vi "Compression.vi"(5 "measure call context in":refnum<class "Measure Call Context.lvclass">, 7 "SMU Settings":T2={"SMU Name"="PXI1Slot15", "SMU Channel"="2", "IDD Current Limit (A)"=0.0}, 8 "error in":errorcluster, 9 "RFmx Settings":T3={"RFmx Name"="5842_0", "RFmx Port"="", "Attenuation"={"Mode"=enum."Constant Attenuation", "Constant Attenuation"={"RFmx External Attenuation (dB)"=1.2}, "s2p File"={"RFmx S-Parameters Orientation"=24000, "RFmx Attenuation s2p File"=path ""}}} {"Attenuation"."s2p File"."RFmx S-Parameters Orientation" items=["Port1 Towards DUT"=24000, "Port2 Towards DUT"=24001]; "Attenuation"."Constant Attenuation"."RFmx External Attenuation (dB)" format="%.2f"}, 10 "RFSG Settings":T4={"RFSG Name"="5842_0", "RFSG Port"="", "Attenuation"={"Mode"=enum."Constant Attenuation", "Contant Attenuation"={"RFSG External Attenuation (dB)"=2.0}, "s2p File"={"RFSG S-parameters Orientation"=24000, "RFSG s2p File Path"=path ""}}} {"Attenuation"."s2p File"."RFSG S-parameters Orientation" items=["Port1 Towards DUT"=24000, "Port2 Towards DUT"=24001]; "Attenuation"."Contant Attenuation"."RFSG External Attenuation (dB)" format="%.2f"}, 11 "Test Configuration":T5={"Expected DUT Gain (dB)"=17.5, "Max Linear Range (dBm)"=-10.0, "Compression Point (dB)"=1.0, "Pout at Pin (dBm)"=1.0, "RFSG Frequency Start (Hz)"=6000000000.0, "RFSG Frequency Stop (Hz)"=18000000000.0, "RFSG Number of Frequency Step"=10, "Power Start (dBm)"=-20.0, "Power Stop(dBm)"=1.0, "Power Step Size (dB)"=4.0, "RBW (Hz)"=5000000.0, "Modes"={"RF Measurement Interval (s)"=0.001, "DC Measurement Interval (s)"=0.0, "Power Stimulus Mode"=enum."Constant Power and RF", "CP_CW_DC Source Delay (s)"=0.0002, "CP_PRF_RF Pulse Width (s)"=0.0009, "CP_PRF_PRI (s)"=0.015, "CP_PRF_DC Source Delay (s)"=0.0, "CP_PRF_RFmx Trigger Delay (s)"=0.2, "PP_PRF_RF Pulse Width (s)"=0.0, "PP_PRF_PRI (s)"=0.0, "PP_PRF_DC Pulse Width (s)"=0.0008, "PP_PRF_Bias Voltage Level (V)"=0.0, "PP_PRF_Bias Current Limit (A)"=0.2, "PP_PRF_DC Source Delay (s)"=0.0, "PP_PRF_RFmx Trigger Delay (s)"=0.0}} {"Pout at Pin (dBm)" format="%#pdBm"; "Modes"."PP_PRF_RFmx Trigger Delay (s)" format="%#ps"; "Modes"."PP_PRF_DC Source Delay (s)" format="%#ps"; "Modes"."PP_PRF_Bias Current Limit (A)" format="%#pA"; "Modes"."PP_PRF_Bias Voltage Level (V)" format="%#pV"; "Modes"."PP_PRF_DC Pulse Width (s)" format="%#ps"; "Modes"."PP_PRF_PRI (s)" format="%#ps"; "Modes"."PP_PRF_RF Pulse Width (s)" format="%#ps"; "Modes"."CP_PRF_RFmx Trigger Delay (s)" format="%#ps"; "Modes"."CP_PRF_DC Source Delay (s)" format="%#ps"; "Modes"."CP_PRF_PRI (s)" format="%#ps"; "Modes"."CP_PRF_RF Pulse Width (s)" format="%#ps"; "Modes"."CP_CW_DC Source Delay (s)" format="%#ps"; "Modes"."DC Measurement Interval (s)" format="%#_6p"; "RFSG Frequency Stop (Hz)" format="%#_6p"; "Power Start (dBm)" format="%#_6p"; "Power Stop(dBm)" format="%#_6p"; "RFSG Frequency Start (Hz)" format="%#_6p"; "Expected DUT Gain (dB)" step=1.0 format="%#_6p"}) -> (0 "error out":errorcluster, 3 "Data":T1)   [LabVIEW 2023]
doc: "This example demonstrates how to use MMICsc API for performing PAE measurements and calibration"
uses:
  Controls/Test Config - Compression.ctl
  Controls/RFSG Config - Compression.ctl
  Controls/RFmx Config - Compression.ctl
  <vilib>/Plug-In SDKs/Measurements/Measure Call Context/Measure Call Context.lvclass
  Controls/SMU Config - Compression.ctl
  Controls/Results - Compression.ctl
  <vilib>/niPAEML/Commit Measurement.vi
  <vilib>/niPAEML/Commit NIDCPower.vi
  <vilib>/niPAEML/PAE Measurement.lvlib
panel:
  out "voltage measurements":dbl[](array[numeric])
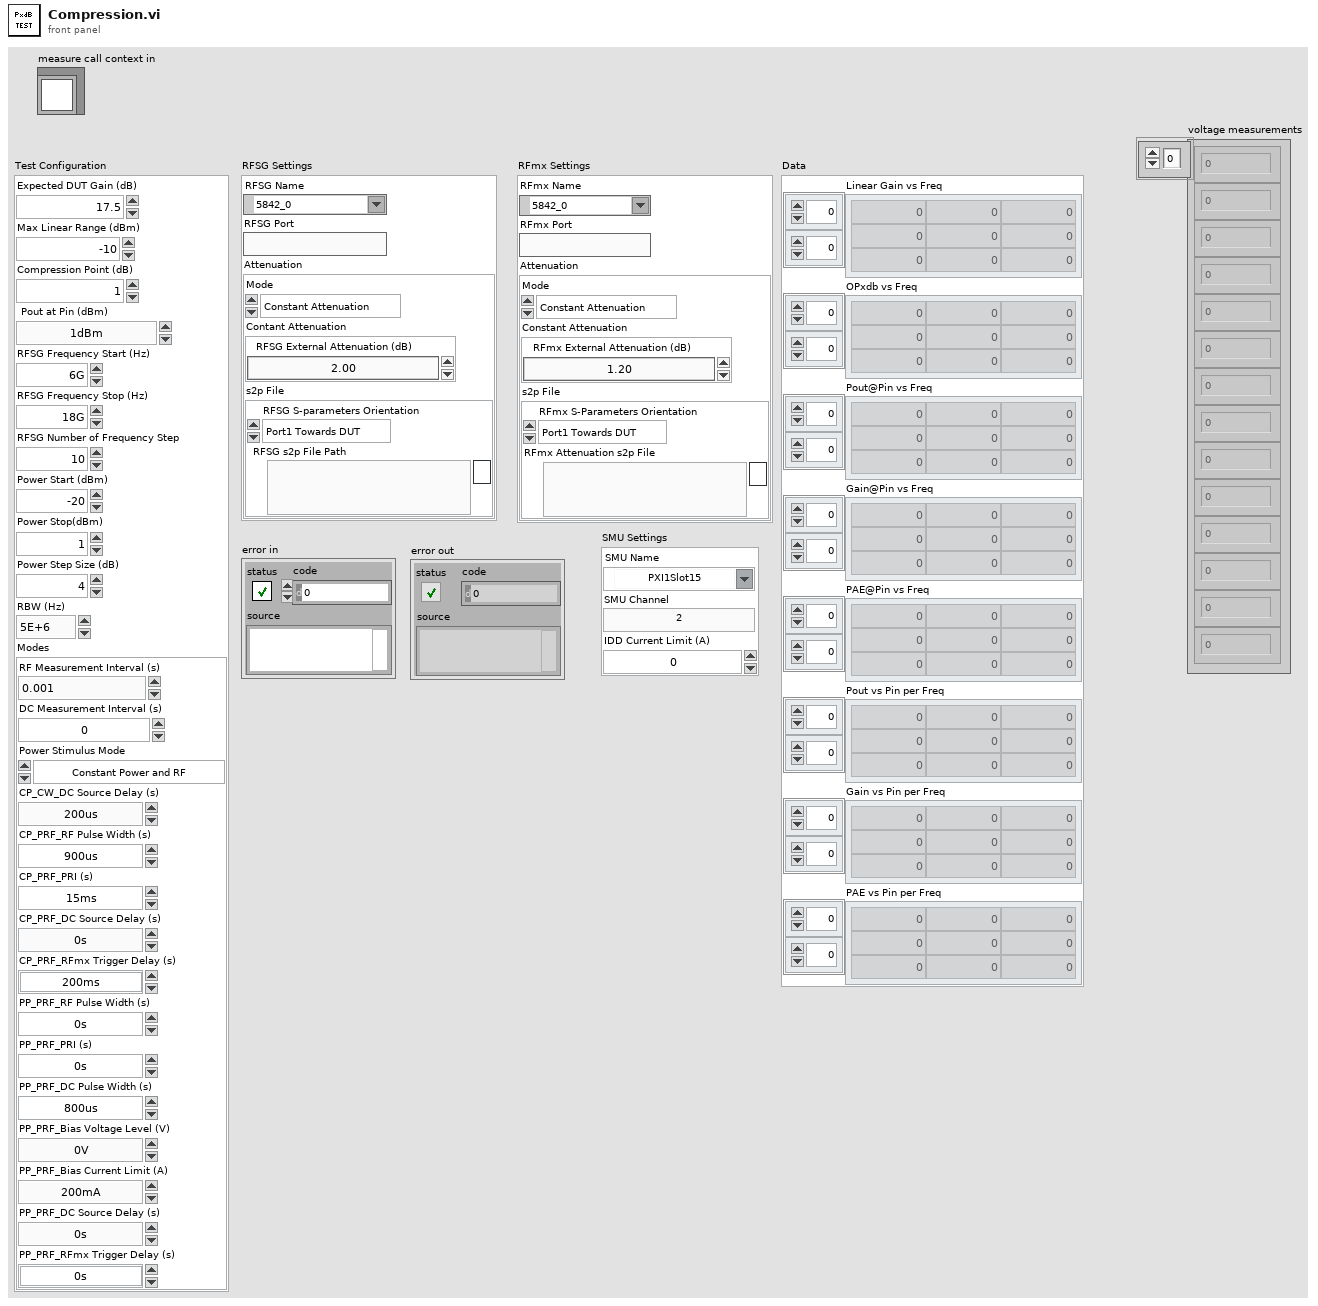
[diagram p1: front panel]
types:
  T1 = typedef "Results - Compression.ctl" = cluster{"Linear Gain vs Freq":dbl[][], "OPxdb vs Freq":dbl[][], "Pout@Pin vs Freq":dbl[][], "Gain@Pin vs Freq":dbl[][], "PAE@Pin vs Freq":dbl[][], "Pout vs Pin per Freq":dbl[][], "Gain vs Pin per Freq":dbl[][], "PAE vs Pin per Freq":dbl[][]}
  T2 = typedef "SMU Config - Compression.ctl" = cluster{"SMU Name":refnum<k15>, "SMU Channel":string, "IDD Current Limit (A)":dbl}
  T3 = typedef "RFmx Config - Compression.ctl" = cluster{"RFmx Name":refnum<k15>, "RFmx Port":string, "Attenuation":cluster{"Mode":enum32{"<None>", "Constant Attenuation", "s2p File"}, "Constant Attenuation":cluster{"RFmx External Attenuation (dB)":dbl}, "s2p File":cluster{"RFmx S-Parameters Orientation":i32, "RFmx Attenuation s2p File":path}}}
  T4 = typedef "RFSG Config - Compression.ctl" = cluster{"RFSG Name":refnum<k15>, "RFSG Port":string, "Attenuation":cluster{"Mode":enum32{"<None>", "Constant Attenuation", "s2p File"}, "Contant Attenuation":cluster{"RFSG External Attenuation (dB)":dbl}, "s2p File":cluster{"RFSG S-parameters Orientation":i32, "RFSG s2p File Path":path}}}
  T5 = typedef "Test Config - Compression.ctl" = cluster{"Expected DUT Gain (dB)":dbl, "Max Linear Range (dBm)":dbl, "Compression Point (dB)":dbl, "Pout at Pin (dBm)":dbl, "RFSG Frequency Start (Hz)":dbl, "RFSG Frequency Stop (Hz)":dbl, "RFSG Number of Frequency Step":i32, "Power Start (dBm)":dbl, "Power Stop(dBm)":dbl, "Power Step Size (dB)":dbl, "RBW (Hz)":dbl, "Modes":cluster{"RF Measurement Interval (s)":dbl, "DC Measurement Interval (s)":dbl, "Power Stimulus Mode":enum16{"Constant Power and RF", "Constant Power and Pulsed RF", "Pulsed Power and RF"}, "CP_CW_DC Source Delay (s)":dbl, "CP_PRF_RF Pulse Width (s)":dbl, "CP_PRF_PRI (s)":dbl, "CP_PRF_DC Source Delay (s)":dbl, "CP_PRF_RFmx Trigger Delay (s)":dbl, "PP_PRF_RF Pulse Width (s)":dbl, "PP_PRF_PRI (s)":dbl, "PP_PRF_DC Pulse Width (s)":dbl, "PP_PRF_Bias Voltage Level (V)":dbl, "PP_PRF_Bias Current Limit (A)":dbl, "PP_PRF_DC Source Delay (s)":dbl, "PP_PRF_RFmx Trigger Delay (s)":dbl}}
  T6 = typedef "PAE Measurement.lvlib/PAE Reference.lvclass/Session Handle.ctl" = refnum<data-value>
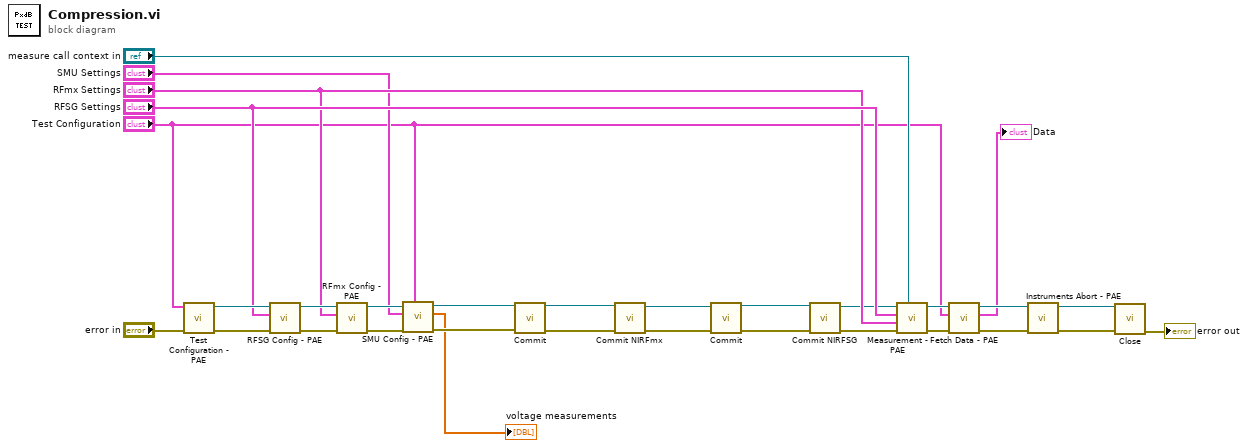
[diagram p0: block diagram]
diagram:
  n1 = call "Test Configuration - PAE.vi"("error in"="error in", "Test Configuration"="Test Configuration") -> ("error out"=w27:errorcluster, "PAE Reference Out"=w30:T6)  [unwired: 7 in, 1 out]
  n2 = call "RFSG Config - PAE.vi"("error in"=w27, "RFSG Settings"="RFSG Settings", "PAE Reference in"=w30) -> ("error out"=w25:errorcluster, "PAE Reference out"=w26:T6)  [unwired: 7 in]
  n3 = call "RFmx Config - PAE.vi"("error in"=w25, "RFmx Settings"="RFmx Settings", "PAE Reference in"=w26) -> ("error out"=w15:errorcluster, "PAE Reference out"=w16:T6)  [unwired: 7 in]
  n4 = call "SMU Config - PAE.vi"("Test Configuration"="Test Configuration", "error in"=w15, "SMU Settings"="SMU Settings", "Data Value Reference in"=w16) -> ("error out"=w14:errorcluster, "voltage measurements"=→"voltage measurements":dbl[], "Data Value Reference out"=w13:T6)  [unwired: 5 in]
  n5 = call-poly <vilib>:"Commit.vi"("PAE Reference In"=w13, "error in"=w14) -> ("PAE Reference Out"=w12:T6, "error out"=w11:errorcluster)  [unwired: 12 in]
  n6 = call "Commit NIRFmx.vi"("error in"=w11, "PAE Reference In"=w12) -> ("error out"=w9:errorcluster, "PAE Reference Out"=w10:T6)  [unwired: 8 in]
  n7 = call-poly <vilib>:"Commit.vi"("PAE Reference In"=w10, "error in"=w9) -> ("PAE Reference Out"=w8:T6, "error out"=w7:errorcluster)  [unwired: 12 in]
  n8 = call "Commit NIRFSG.vi"("error in"=w7, "PAE Reference In"=w8) -> ("error out"=w5:errorcluster, "PAE Reference Out"=w6:T6)  [unwired: 8 in]
  n9 = call "Measurement - PAE.vi"("measure call context in"="measure call context in", "error in"=w5, "RFmx Settings"="RFmx Settings", "RFSG Settings"="RFSG Settings", "PAE Reference in"=w6) -> ("error out"=w28:errorcluster, "PAE Reference out"=w24:T6)  [unwired: 5 in]
  n10 = call "Fetch Data - PAE.vi"("error in"=w28, "Test Configuration"="Test Configuration", "PAE Reference in"=w24) -> ("error out"=w19:errorcluster, "Data"=→"Data":T1, "PAE Reference out"=w20:T6)  [unwired: 6 in]
  n11 = call "Instruments Abort - PAE.vi"("error in"=w19, "PAE Reference in"=w20) -> ("error out"=w17:errorcluster, "PAE Reference Out"=w18:T6)  [unwired: 8 in]
  n12 = call <vilib>:"Close.vi"("PAE Reference In"=w18, "error in"=w17) -> ("error out"=→"error out":errorcluster)  [unwired: 13 in]
